vi "DriverStationGetInstructions.vi"   [LabVIEW 2018]
uses:
  <vilib>/Rock Robotics/Network Tables/NT Read Number.vi
  instructions.vi
  refnums.vi
  <vilib>/Rock Robotics/WPI/Utilities/WPI_GetSetVariantRefNum.vi
types:
  T1 = typedef "WPI_JoystickDevRef.ctl" = cluster{"Device":T2}
  T2 = typedef "WPI_JoystickDeviceEnum.ctl" = enum16{"USB 0", "USB 1", "USB 2", "USB 3", "USB 4", "USB 5"}
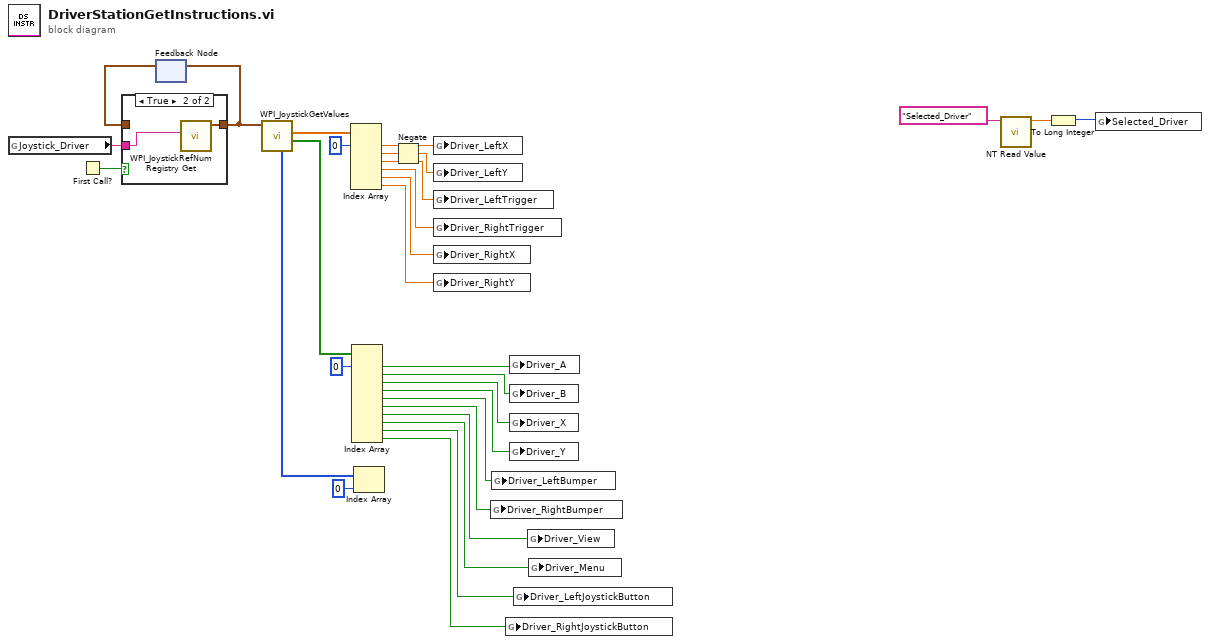
[diagram p0: block diagram]
diagram:
  n1 = global read "refnums.vi" "Joystick_Driver"() -> (w27:string)
  n2 = First Call?() -> (First Call?: T/F=w30:bool)
  n3 = feedback #1() -> (w29:T1)  [unwired: 1 in]
  n4 = case shown="True" w30 {
    tunnel: [w31 w33] -> w28
    tunnel: w29 -> [w31 _]
    tunnel: w27 -> [_ w32]
    frame False {
    }
    frame True {
      n5 = call <vilib>:"WPI_JoystickRefNum Registry Get.vi"("refnum name"=w32) -> ("JoystickDevRef"=w33:T1)  [unwired: 9 in, 1 out]
    }
  }
  n6 = feedback-in #1(w28) -> ()
  n7 = call <vilib>:"WPI_JoystickGetValues.vi"("JoystickDevRef"=w28) -> ("Buttons"=w25:bool[], "Axes"=w26:dbl[], "POVs"=w22:i16[])  [unwired: 6 in, 2 out]
  n8 = Index Array(array=w26, index #1=0 ("index")) -> (element #1=w10:dbl, element #2=w9:dbl, element #3=w8:dbl, element #4=w7:dbl, element #5=w6:dbl, element #6=w5:dbl)  [unwired: 5 in]
  n9 = Index Array(array=w25, index #1=0 ("index")) -> (element #1=w20:bool, element #2=w19:bool, element #3=w18:bool, element #4=w17:bool, element #5=w16:bool, element #6=w15:bool, element #7=w14:bool, element #8=w13:bool, element #9=w12:bool, element #10=w11:bool)  [unwired: 9 in]
  n10 = Index Array(array=w22, index=0) -> ()  [unwired: 1 out]
  n11 = Negate(x=w9) -> (-x=w1:dbl)
  n12 = global write "instructions.vi" "Driver_LeftX"(w10) -> ()
  n13 = global write "instructions.vi" "Driver_LeftY"(w1) -> ()
  n14 = global write "instructions.vi" "Driver_LeftTrigger"(w8) -> ()
  n15 = global write "instructions.vi" "Driver_RightTrigger"(w7) -> ()
  n16 = global write "instructions.vi" "Driver_RightX"(w6) -> ()
  n17 = global write "instructions.vi" "Driver_RightY"(w5) -> ()
  n18 = global write "instructions.vi" "Driver_RightBumper"(w15) -> ()
  n19 = global write "instructions.vi" "Driver_LeftBumper"(w16) -> ()
  n20 = global write "instructions.vi" "Driver_RightJoystickButton"(w11) -> ()
  n21 = global write "instructions.vi" "Driver_A"(w20) -> ()
  n22 = global write "instructions.vi" "Driver_B"(w19) -> ()
  n23 = global write "instructions.vi" "Driver_X"(w18) -> ()
  n24 = global write "instructions.vi" "Driver_Y"(w17) -> ()
  n25 = global write "instructions.vi" "Driver_LeftJoystickButton"(w12) -> ()
  n26 = global write "instructions.vi" "Driver_View"(w14) -> ()
  n27 = global write "instructions.vi" "Driver_Menu"(w13) -> ()
  n28 = call-poly <vilib>:"NT Read Value.vi"("Name"="Selected_Driver" ("refnum name")) -> ("Numeric"=w3:dbl)  [unwired: 9 in, 1 out]
  n29 = To Long Integer(number=w3) -> (32bit integer=w2:i32)
  n30 = global write "instructions.vi" "Selected_Driver"(w2) -> ()
